vi "Write JoystickDevRef.vi"(8 "error in (no error)":errorcluster, 10 "JoystickDevRef":T1, 11 "XBoxController in":refnum<class "XBoxController.lvclass">) -> (0 "error out":errorcluster, 3 "XBoxController out":refnum<class "XBoxController.lvclass">)   [LabVIEW 2013, in "XBoxController.lvclass"]
uses:
  XBoxController.lvclass
  <vilib>/Rock Robotics/WPI/Joystick/WPI_JoystickDevRef.ctl
  <vilib>/Rock Robotics/WPI/Joystick/WPI_JoystickDeviceEnum.ctl
  XBoxController.lvclass/XBoxController.ctl
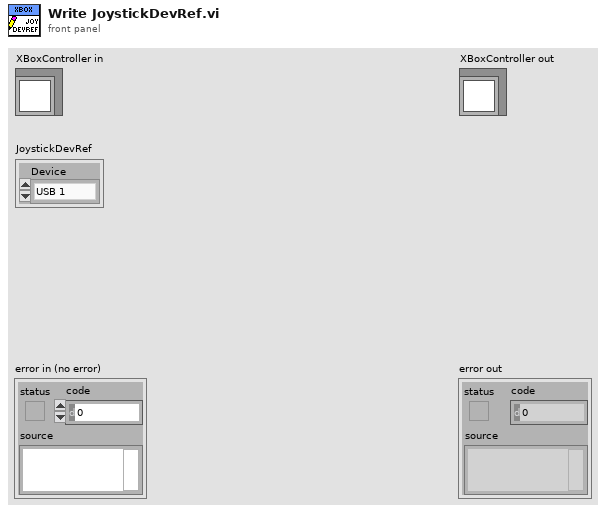
[diagram p1: front panel]
types:
  T1 = typedef "WPI_JoystickDevRef.ctl" = cluster{"Device":T2}
  T2 = typedef "WPI_JoystickDeviceEnum.ctl" = enum16{"USB 1", "USB 2", "USB 3", "USB 4", "Kinect 1", "Kinect 2"}
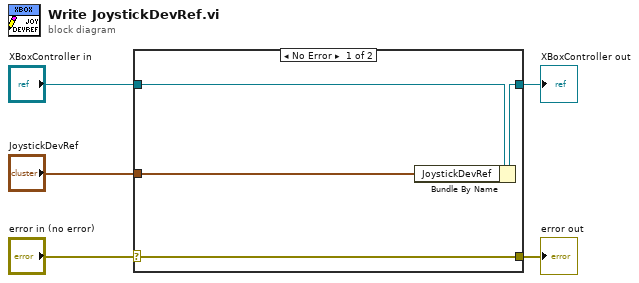
[diagram p0: block diagram]
diagram:
  n1 = case shown="No Error" "error in (no error)" {
    selector: "error in (no error)" -> [w9 w10]
    tunnel: [w9 w10] -> w4
    tunnel: [w7 w11] -> w2
    tunnel: "XBoxController in" -> [w8 w11]
    tunnel: "JoystickDevRef" -> [w6 _]
    frame No Error {
      n2 = Bundle By Name(cluster=w8, "JoystickDevRef"=w6) -> (w7:refnum<class "XBoxController.lvclass">)
    }
    frame Error {
    }
  }
  "error out" <- w4
  "XBoxController out" <- w2
